vi "Quit.vi"(8 "error in (no error)":errorcluster, 11 "Engine in":refnum<class "Engine.lvclass">) -> (0 "error out":errorcluster)   [LabVIEW 2024, in "GLF.lvlib" / "Engine.lvclass"]
uses:
  Engine.lvclass
  Command--enum.ctl
  Engine.lvclass/Engine.ctl
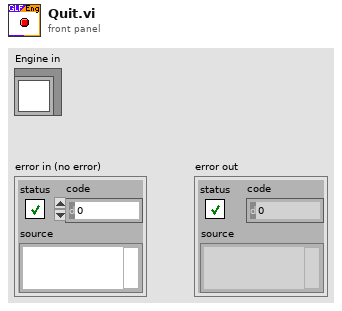
[diagram p1: front panel]
types:
  T1 = typedef "GLF.lvlib/Engine.lvclass/Command--enum.ctl" = enum16{"Quit"}
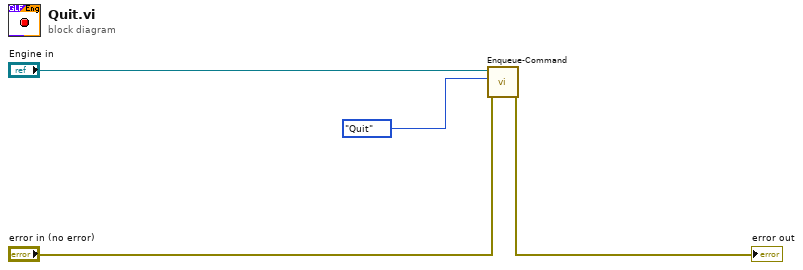
[diagram p0: block diagram]
diagram:
  n1 = call "Enqueue-Command.vi"("error in (no error)"="error in (no error)", "Cmd"=Command--enum."Quit", "Engine in"="Engine in") -> ("error out"=→"error out":errorcluster)  [unwired: 6 in, 2 out]
